vi "Manual Override.vi"(8 "Override":T1, 10 "Enable":bool, 11 "Auto CMD":T2) -> (3 "OverRide Command Out":T2)   [LabVIEW 2023, in "Template FX_ACT.lvlib"]
uses:
  Template FX_ACT.lvlib
  Cluster_CMD_ACT_Data.ctl
  ENUM_CMD_Mode Select.ctl
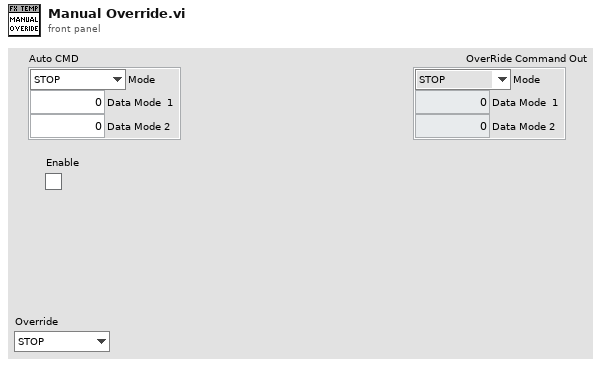
[diagram p1: front panel]
types:
  T1 = typedef "Template FX_ACT.lvlib/ENUM_CMD_Mode Select.ctl" = enum16{"STOP", "Mode 1", "Mode 2"}
  T2 = typedef "Template FX_ACT.lvlib/Cluster_CMD_ACT_Data.ctl" = cluster{"Mode":T1, "Data Mode  1":dbl, "Data Mode 2":dbl}
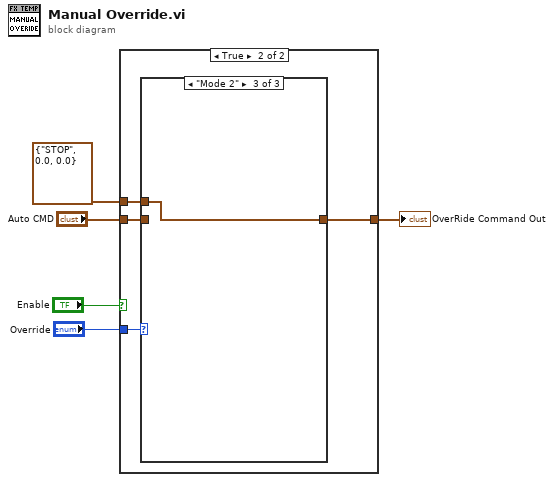
[diagram p0: block diagram]
diagram:
  n1 = case shown="True" "Enable" {
    tunnel: [w6 w10] -> w5
    tunnel: "Auto CMD" -> [w6 w9]
    tunnel: T2 {"Mode"=enum."STOP", "Data Mode  1"=0.0, "Data Mode 2"=0.0} ("OverRide Command Out") -> [_ w8]
    tunnel: "Override" -> [_ w7]
    frame False {
    }
    frame True {
      n2 = case shown="\"Mode 2\"" w7 {
        tunnel: [w11 w12 w13] -> w10
        tunnel: w8 -> [w11 w12 w13]
        tunnel: w9 -> [_ _ _]
        frame "STOP" {
        }
        frame "Mode 1" {
        }
        frame "Mode 2" {
        }
      }
    }
  }
  "OverRide Command Out" <- w5
